vi "Get Status.vi"(8 "error in (no error)":errorcluster caption="entrée d'erreur (pas d'erreur)", 11 "Class Shielding_ Box en entrée":refnum<class "Class Shielding_ Box JC-PB3044.lvclass">) -> (0 "error out":errorcluster caption="sortie d'erreur", 3 "Class Shielding_ Box en sortie":refnum<class "Class Shielding_ Box JC-PB3044.lvclass">)   [LabVIEW 2020, in "Library Instrument & Equipement.lvlib" / "Library Shielding box.lvlib" / "Class Shielding_ Box JC-PB3044.lvclass"]
uses:
  Class Shielding_ Box JC-PB3044.lvclass
  C:/Users/ngarcin/OneDrive - Altyor/Standard TB/Class/Shielding box/Class Shielding box (Default)/Class Shielding_ Box (Default).lvclass
  Class Shielding_ Box JC-PB3044.lvclass/Class Shielding_ Box JC-PB3044.ctl
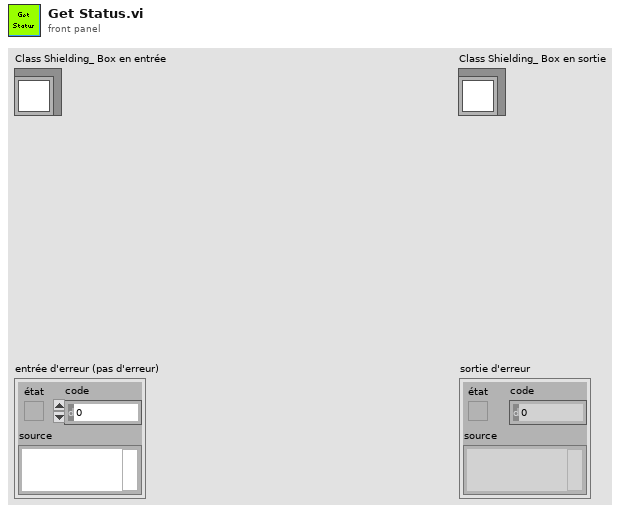
[diagram p1: front panel]
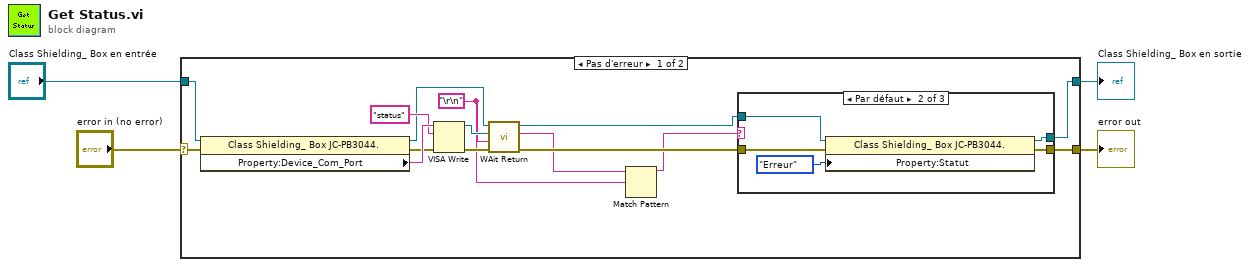
[diagram p0: block diagram]
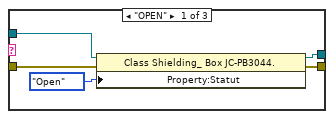
[diagram p2: hidden frame]
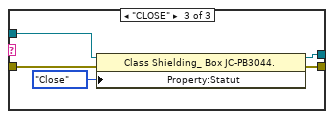
[diagram p3: hidden frame]
diagram:
  n1 = case shown="Pas d'erreur" "error in (no error)" {
    selector: "error in (no error)" -> [w16 w36]
    tunnel: [w8 w36] -> w2
    tunnel: [w10 w35] -> w1
    tunnel: "Class Shielding_ Box en entrée" -> [w19 w35]
    frame No Error {
      w7 = "\r\n"
      n2 = property class="Class Shielding_ Box JC-PB3044."(reference=w19, error in=w16) -> (reference out=w12:refnum<class "Class Shielding_ Box JC-PB3044.lvclass">, error out=w15:errorcluster, "Property:Device_Com_Port"=w18:string)
      n3 = VISA Write(VISA resource name=w18, write buffer="status" ("buffer d'écriture"), error in (no error)=w15) -> (VISA resource name out=w14:refnum<visa-resource-name>, error out=w13:errorcluster)  [unwired: 1 out]
      n4 = call "WAit Return.vi"("entrée d'erreur (pas d'erreur)"=w13, "String Wait"=w7, "VISA resource name"=w14, "Class Shielding_ Box JC-PB3044 en entrée"=w12) -> ("sortie d'erreur"=w9:errorcluster, "Frame receive"=w6:string, "Class Shielding_ Box JC-PB3044 en sortie"=w11:refnum<class "Class Shielding_ Box JC-PB3044.lvclass">)  [unwired: 5 in]
      n5 = Match Pattern(string=w6, regular expression=w7) -> (before substring=w5:string)  [unwired: 1 in, 3 out]
      n6 = case shown="Par défaut" w5 {
        tunnel: w11 -> [w24 w29 w34]
        tunnel: [w23 w28 w33] -> w10
        tunnel: w9 -> [w22 w27 w32]
        tunnel: [w21 w26 w31] -> w8
        frame "OPEN" {
          n7 = property class="Class Shielding_ Box JC-PB3044."(reference=w24, error in=w22, "Property:Statut"=enum16{"Erreur", "Close", "Open"}."Open" ("Statut")) -> (reference out=w23:refnum<class "Class Shielding_ Box JC-PB3044.lvclass">, error out=w21:errorcluster)
        }
        frame Default {
          n8 = property class="Class Shielding_ Box JC-PB3044."(reference=w29, error in=w27, "Property:Statut"=enum16{"Erreur", "Close", "Open"}."Erreur" ("Statut")) -> (reference out=w28:refnum<class "Class Shielding_ Box JC-PB3044.lvclass">, error out=w26:errorcluster)
        }
        frame "CLOSE" {
          n9 = property class="Class Shielding_ Box JC-PB3044."(reference=w34, error in=w32, "Property:Statut"=enum16{"Erreur", "Close", "Open"}."Close" ("Statut")) -> (reference out=w33:refnum<class "Class Shielding_ Box JC-PB3044.lvclass">, error out=w31:errorcluster)
        }
      }
    }
    frame Error {
    }
  }
  "error out" <- w2
  "Class Shielding_ Box en sortie" <- w1
